vi "Matrix_ExtractFrom.vi"(8 "other":T1, 9 "StartingColumn":i32, 10 "StartingRow":i32, 11 "input matrix":T1) -> (3 "output column":T1)   [LabVIEW 2019, in "Trajectory_Library.lvlib"]
doc: "Extracts a submatrix from the supplied matrix and inserts it in a submatrix in \"this\". The shape of \"this\" is used to determine the size of the matrix extracted.\n \nInputs:\n - input matrix -- The input matrix\n - startingRow -- The starting row in the supplied matrix to extract the submatrix.\n - startingCol -- The starting column in the supplied matrix to extract the submatrix.\n - other -- The matrix to extract the submatrix from.\n\n\nOutputs:\n - output column -- the column matrix resulting from the extraction"
uses:
  Trajectory_Library.lvlib
  <vilib>/Analysis/Matrix/Datatypes/RealMatrix.ctl
  <vilib>/Analysis/Matrix/NI_Matrix.lvlib
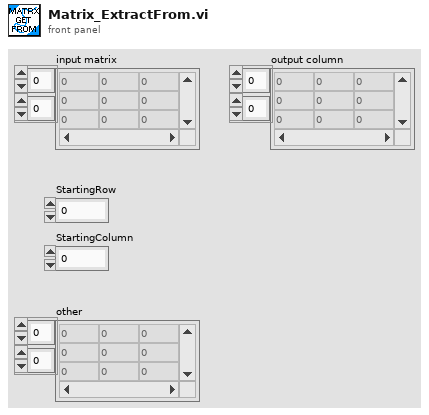
[diagram p1: front panel]
types:
  T1 = typedef "NI_Matrix.lvlib/RealMatrix.ctl" = dbl[][]
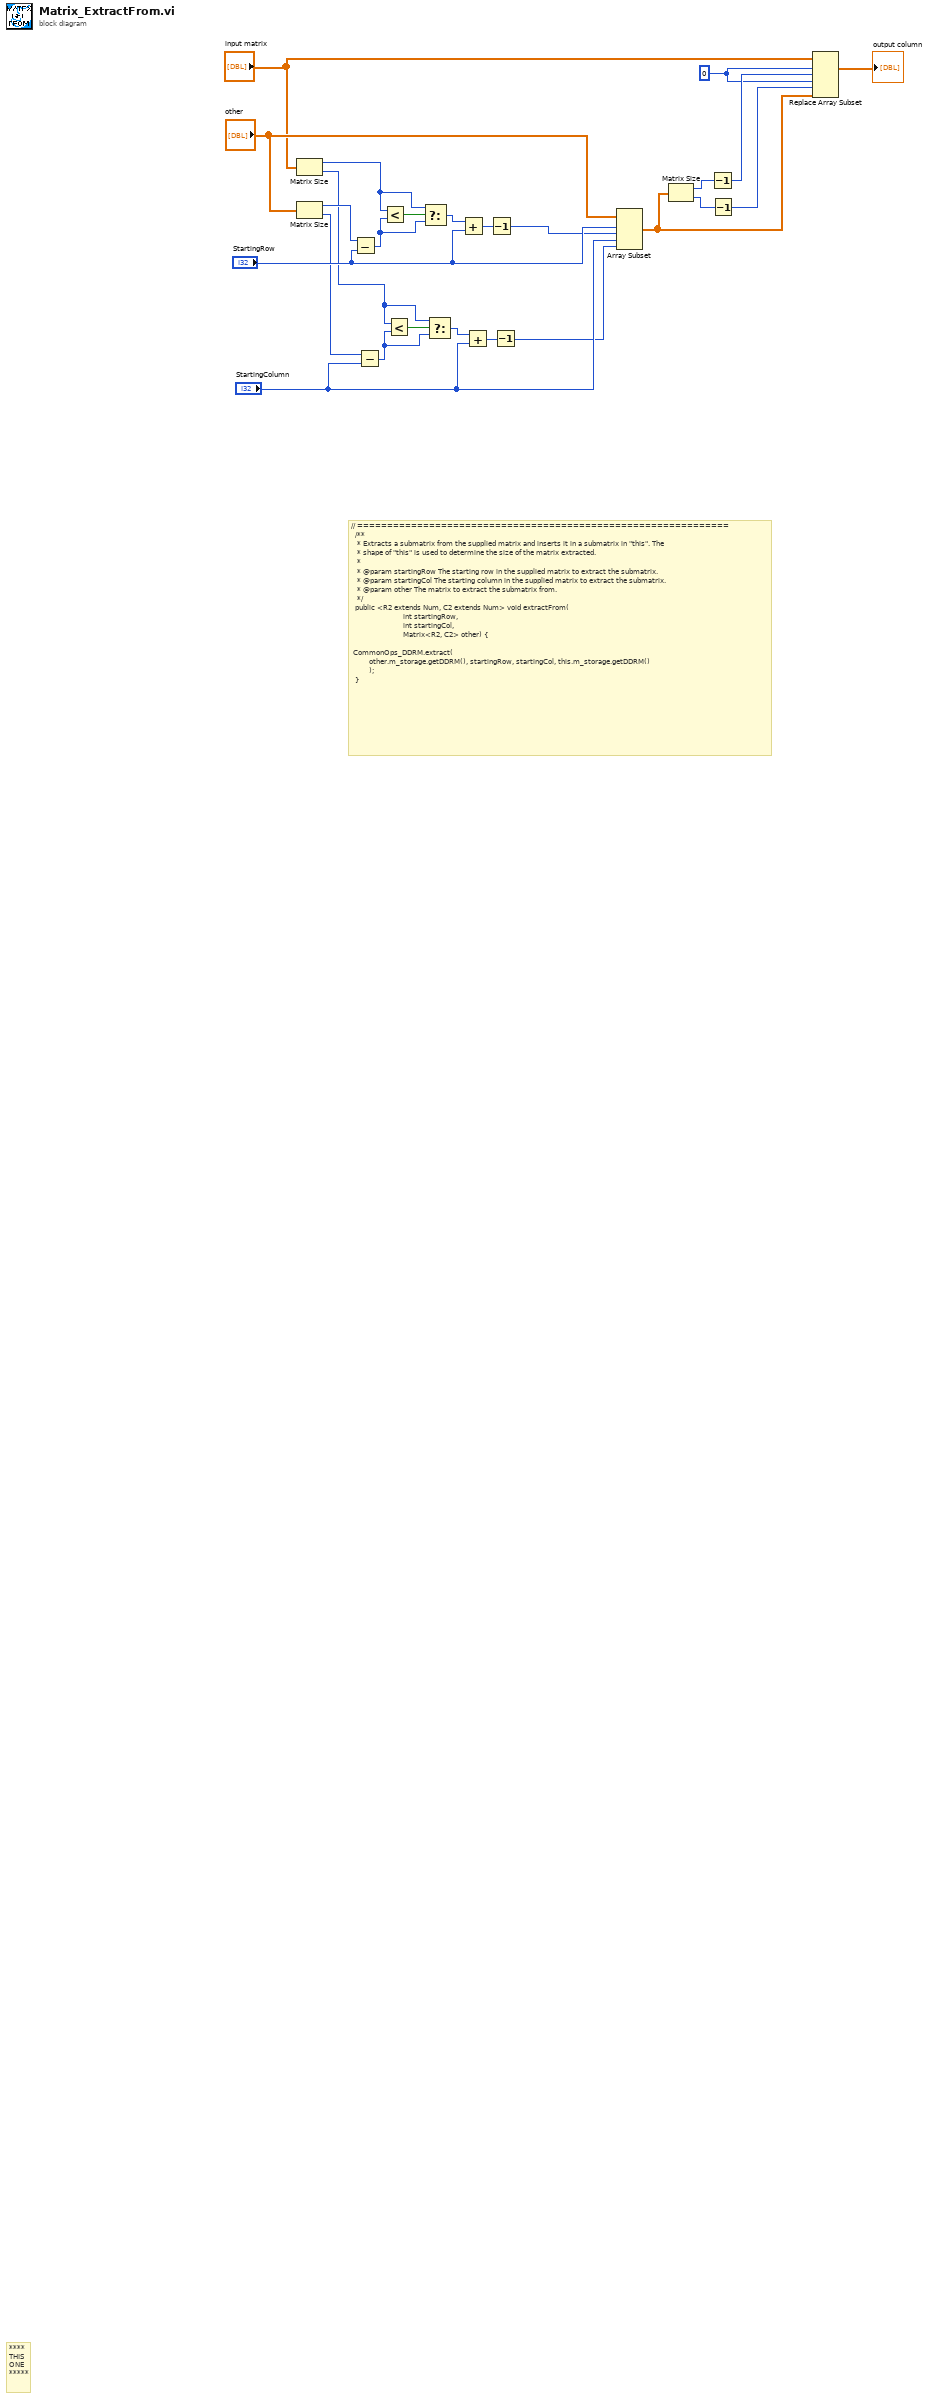
[diagram p0: block diagram]
diagram:
  w4 = 0 ("row 1")
  # "// ==============================================================\n  /**\n   * Extracts a submatrix from the supplied matrix and inserts it in a submatrix in \"this\". The\n   * shape of \"this\" is used to determine the size of the matrix extracted.\n   *\n   * @param startingRow The starting row in the supplied matrix to extract the submatrix.\n   * @param startingCol The starting column in the supplied matrix to extract the submatrix.\n   * @param other The matrix to extract the submatrix from.\n   */\n  public <R2 extends Num, C2 extends Num> void extractFrom(\n      \t\t                  int startingRow, \n\t\t                        int startingCol, \n\t\t                        Matrix<R2, C2> other) {\n    \n\tCommonOps_DDRM.extract(\n        \tother.m_storage.getDDRM(), startingRow, startingCol, this.m_storage.getDDRM()\n         );\n  }"
  # "****\nTHIS\nONE\n*****"
  n1 = Matrix Size(0:"input matrix") -> (1:w2:i32, 2:w1:i32)
  n2 = Matrix Size(0:"other") -> (1:w24:i32, 2:w13:i32)
  n3 = Subtract(x=w24, y="StartingRow") -> (x-y=w22:i32)
  n4 = Subtract(x=w13, y="StartingColumn") -> (x-y=w16:i32)
  n5 = Less?(x=w2, y=w22) -> (x < y?=w23:bool)
  n6 = Less?(x=w1, y=w16) -> (x < y?=w17:bool)
  n7 = Select(t=w2, s=w23, f=w22) -> (s? t:f=w21:i32)
  n8 = Select(t=w1, s=w17, f=w16) -> (s? t:f=w15:i32)
  n9 = Add(x=w21, y="StartingRow") -> (x+y=w19:i32)
  n10 = Add(x=w15, y="StartingColumn") -> (x+y=w14:i32)
  n11 = Decrement(x=w19) -> (x-1=w18:i32)
  n12 = Decrement(x=w14) -> (x-1=w11:i32)
  n13 = Array Subset(array="other", index (row)="StartingRow", length (row)=w18, index (col)="StartingColumn", length (col)=w11) -> (w8:T1)
  n14 = Matrix Size(0:w8) -> (1:w6:i32, 2:w7:i32)
  n15 = Decrement(x=w6) -> (x-1=w5:i32)
  n16 = Decrement(x=w7) -> (x-1=w3:i32)
  n17 = Replace Array Subset(array="input matrix", new element=w8, index (dim 0)=w4, index (dim 1)=w5, index (dim 2)=w4, index (dim 3)=w3) -> (→"output column":T1)
